vi "Pose_getTranslation.vi"(11 "in POSE":T2) -> (3 "outTRANSLATION":T1)   [LabVIEW 2019, in "Trajectory_Library.lvlib"]
doc: "Returns the translation component of the transformation.\n\nParmeters:\n- IN POSE - The POSE data structure\n\nRETURNS:\n - OUT TRANSLATION - The translational component of the pose."
uses:
  Trajectory_Library.lvlib
  POSE2D.ctl
  TRANSLATION2D.ctl
  ROTATION2D.ctl
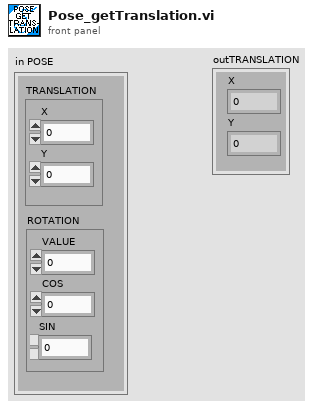
[diagram p1: front panel]
types:
  T1 = typedef "Trajectory_Library.lvlib/TRANSLATION2D.ctl" = cluster{"X":dbl, "Y":dbl}
  T2 = typedef "Trajectory_Library.lvlib/POSE2D.ctl" = cluster{"TRANSLATION":T1, "ROTATION":T3}
  T3 = typedef "Trajectory_Library.lvlib/ROTATION2D.ctl" = cluster{"VALUE":dbl, "COS":dbl, "SIN":dbl}
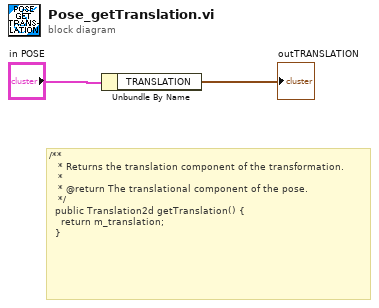
[diagram p0: block diagram]
diagram:
  # "/**\n   * Returns the translation component of the transformation.\n   *\n   * @return The translational component of the pose.\n   */\n  public Translation2d getTranslation() {\n    return m_translation;\n  }"
  n1 = Unbundle By Name("in POSE") -> ("TRANSLATION"=→"outTRANSLATION":T1)
